vi "Parse Core.vi"(8 "error in (no error)":errorcluster, 11 "Config Parser BML in":refnum<class "Config Parser BML.lvclass">) -> (0 "error out":errorcluster, 2 "Config Array":string[](array[string]), 3 "Config Parser BML out":refnum<class "Config Parser BML.lvclass">)   [LabVIEW 2018, in "Config Parser BML.lvlib" / "Config Parser BML.lvclass"]
uses:
  Config Parser BML.lvclass
  C:/P4 Workspace/PC Client/Solutions/5g_eap/trunk/1.0/HiSi5GmmWave/Pattern_Gen_Tool/Interfaces/File Parser Interface.lvlibp/Interfaces/File Parser Interface/File Parser Interface.lvclass
  Interfaces/File Parser Interface.lvlibp/Interfaces/File Parser Interface/Read File Path.vi
  <vilib>/Utility/file.llb/Read Delimited Spreadsheet (string).vi
  Interfaces/File Parser Interface.lvlibp/Interfaces/File Parser Interface/File Parser Interface.lvclass
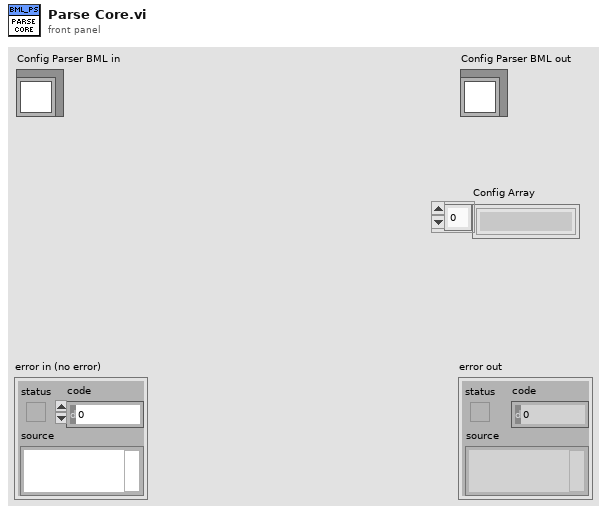
[diagram p1: front panel]
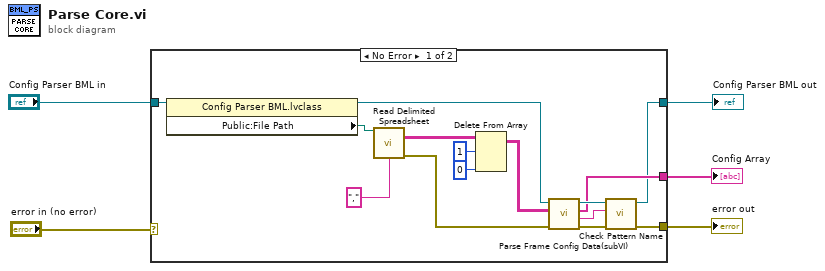
[diagram p0: block diagram]
diagram:
  n1 = case shown="No Error" "error in (no error)" {
    selector: "error in (no error)" -> [_ w21]
    tunnel: "Config Parser BML in" -> [w20 w22]
    tunnel: [w9 _] -> w3
    tunnel: [w8 w21] -> w2
    tunnel: [w7 w22] -> w1
    frame No Error {
      n2 = property class="Config Parser BML.lvclass"(reference=w20) -> (reference out=w14:refnum<class "Config Parser BML.lvclass">, "Public:File Path"=w6:path)  [unwired: 1 in, 1 out]
      n3 = call-poly <vilib>:"Read Delimited Spreadsheet.vi"("file path (dialog if empty)"=w6, "delimiter (\\t)"="," ("delimiter (\\t)")) -> ("all rows"=w19:string[][], "error out"=w13:errorcluster)  [unwired: 8 in, 4 out]
      n4 = Delete From Array(array=w19, length=1, index (row)=0) -> (array with subset deleted=w15:string[][])  [unwired: 1 in, 1 out]
      n5 = call-dynamic "Parse Frame Config Data(subVI).vi"("error in (no error)"=w13, "all rows"=w15, "Config Parser BML in"=w14) -> ("error out"=w10:errorcluster, "Pattern Name out"=w11:string, "Config Data"=w9:string[], "Config Parser BML out"=w12:refnum<class "Config Parser BML.lvclass">)  [unwired: 5 in]
      n6 = call "Check Pattern Name.vi"("error in (no error)"=w10, "Pattern Name"=w11, "File Parser Interface in"=w12) -> ("error out"=w8:errorcluster, "File Parser Interface out"=w7:refnum<class "Config Parser BML.lvclass">)  [unwired: 7 in]
    }
    frame Error {
    }
  }
  "error out" <- w2
  "Config Parser BML out" <- w1
  "Config Array" <- w3
